vi "_RT Process Runtime Update.vi"(8 "Error In":errorcluster, 9 "Acquiring Data":bool, 10 "binary string":string, 11 "Command":T1) -> (0 "Error Out":errorcluster)   [LabVIEW 2015]
uses:
  Type/_RT Command.ctl
  Type/_RT Active Ch.ctl
  Type/_RT Parameter.ctl
  Type/_RT Expt.ctl
  Type/_Run Mode.ctl
  Type/_RT Mass Range.ctl
  Type/_RT Res Type.ctl
  _RT Global.vi
  <vilib>/Utility/error.llb/Error Cluster From Error Code.vi
  <vilib>/rvi/errors/niLvFpgaAdjustHostInterfaceError.vi
  <vilib>/rvi/interface/nirviReadWriteControl/nirviReadWriteControl.xnode
  Type/FPGA Typedef.ctl
  FPGA Bitfiles/FPGA9607.lvbitx
  NiFpgaLv.dll
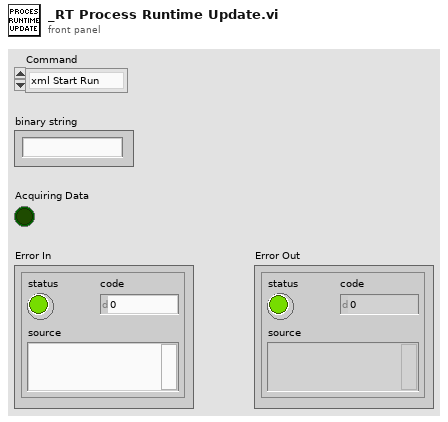
[diagram p1: front panel]
types:
  T1 = typedef "_RT Command.ctl" = enum16{"xml Start Run", "xml Start Actual Run", "xml Stop Run", "xml Runtime Update", "xml Get Status", "xml Get Table", "xml Set Table", "xml Get Configuration", "xml System Status", "xml Set LC Input Logic", "xml Get Data", "xml Get Info", "Start", "StartActualRun", "Stop", "Runtime Update", "Get Data", "Get Info", "Get Status", "Get Param", "Get Config", "Get Table", "Read ADC", "Set Oscillator", "Update Config", "Update Table", "Set All Pol", "Set Pol and DC", "Set Max Mass", "Toggle RP", "Toggle EL", "Set PIC", "Initialize Turbo", "Send Turbo Comm", "Close Turbo", "P1", "P2", "P3", "Send Serial", "Set LC Out", "Get LC In", "Read VAC", "Test Table", "Toggle Power", "Get Startup", "Set Startup", "Get ADC Table", "Set ADC Table", "Get Brief Status", "Get Detail Status", "Auxiliary Update", "Set CC Logics", "Set CC Input Logics", "Ignore Error", "invalid"}
  T2 = typedef "_RT Expt.ctl" = cluster{"StartT(mS)":i32, "#Cycles":i32, "Scan Type":T3, "PauseT(uS)":i32, "Polarity":u8, "DelayT(mS)":i32, "Active Ch":T4[], "Mass Range":T5[]}
  T3 = typedef "_Run Mode.ctl" = enum16{"MRM (Q1/Q2)", "Q1 Scan", "Q1 SRM", "Q2 Scan", "Q2 SRM", "Product Scan", "Precursor Scan", "Neutral Loss", "Neutral Gain"}
  T4 = typedef "_RT Active Ch.ctl" = cluster{"Start":i32, "Step":i32, "ChID":i32}
  T5 = typedef "_RT Mass Range.ctl" = cluster{"Steps":i32, "Dwell(uS)":i32, "Resolution Type":T6, "Ramping Ch":T4[]}
  T6 = typedef "_RT Res Type.ctl" = u16
  T7 = typedef "_RT Parameter.ctl" = cluster{"RunMode":i32, "Initial Ch":T4[], "Sync":u8, "Expt":T2[], "EqTime(mS)":i32}
  T8 = typedef "_RT Instrument State.ctl" = enum16{"Initializing", "Mass Spectrometer is Off", "Starting Up", "Turning Power Off", "Going to Standby", "Roughing Pump Ready", "Turning Turbo Off", "Turbo Startup", "Turbopump Ready", "Checking Vacuum", "Going to Ready", "Ready", "Running", "Source Standby", "Lost Communication", "Shutting Down", "Fault", "24V Standby", "Go to 24V Standby", "Turbopump Ready-Waiting"}
  T9 = typedef "Semaphore RefNum" = refnum<k1>
  T10 = typedef "_XML Lens.ctl" = cluster{"Value":dbl, "ChID":u8}
  T11 = typedef "FPGA Typedef.ctl" = refnum<k20>
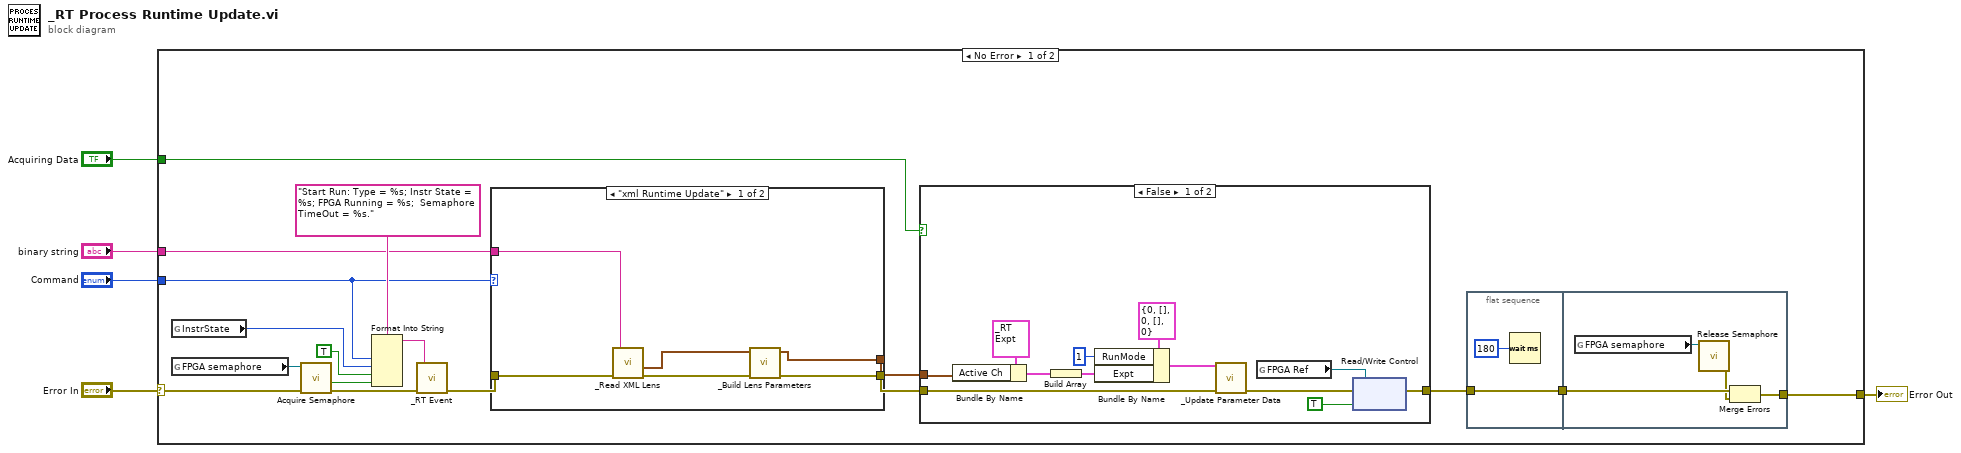
[diagram p0: block diagram]
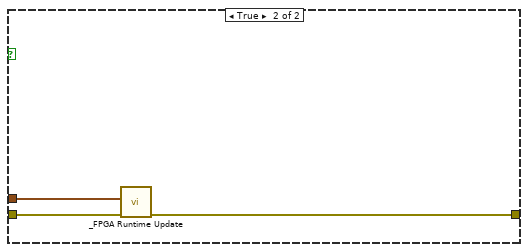
[diagram p2: hidden frame]
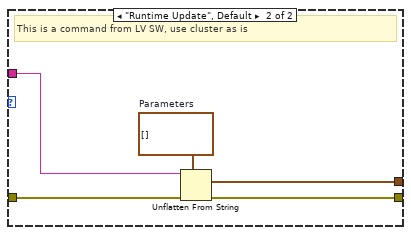
[diagram p3: hidden frame]
diagram:
  n1 = case shown="No Error" "Error In" {
    selector: "Error In" -> [w21 w55]
    tunnel: [w20 w55] -> w4
    tunnel: "Command" -> [w13 _]
    tunnel: "binary string" -> [w12 _]
    tunnel: "Acquiring Data" -> [w6 _]
    frame No Error {
      n2 = global read "_RT Global.vi" "InstrState"() -> (w8:T8)
      n3 = global read "_RT Global.vi" "FPGA semaphore"() -> (w16:T9)
      n4 = call <vilib>:"Acquire Semaphore.vi"("error in (no error)"=w21, "semaphore"=w16) -> ("error out"=w15:errorcluster, "timed out"=w17:bool)  [unwired: 1 in, 3 out]
      n5 = Format Into String(format string="Start Run: Type = %s; Instr State = %s; FPGA Running = %s;  Semaphore TimeOut = %s.", w13, w8, TRUE ("timed out"), w17) -> (resulting string=w18:string)  [unwired: 2 in, 1 out]
      n6 = call "_RT Event.vi"("error in (no error)"=w15, "Event"=w18) -> ("error out"=w14:errorcluster)  [unwired: 1 in, 4 out]
      n7 = case shown="\"xml Runtime Update\"" w13 {
        tunnel: [w46 w53] -> w11
        tunnel: w14 -> [w49 w54]
        tunnel: w12 -> [w48 w52]
        tunnel: [w44 w50] -> w10
        frame "xml Runtime Update" {
          n8 = call "_Read XML Lens.vi"("error in"=w49, "XML String"=w48) -> ("error out"=w47:errorcluster, "Lens"=w45:T10[])  [unwired: 4 out]
          n9 = call "_Build Lens Parameters.vi"("error in"=w47, "Lens"=w45) -> ("error out"=w46:errorcluster, "Array"=w44:T4[])  [unwired: 8 in]
        }
        frame "Runtime Update", Default {
          w51 = T4[] []  # Parameters
          # "This is a command from LV SW, use cluster as is"
          n10 = Unflatten From String(type=w51, binary string=w52, error in (no error)=w54) -> (value=w50:T4[], error out=w53:errorcluster)  [unwired: 3 out]
        }
      }
      n11 = case shown="False" w6 {
        tunnel: w11 -> [w27 w37]
        tunnel: w10 -> [w29 w36]
        tunnel: [w23 w35] -> w9
        frame False {
          n12 = Bundle By Name(cluster=T2 {"StartT(mS)"=0, "#Cycles"=0, "Scan Type"=enum."MRM (Q1/Q2)", "PauseT(uS)"=0, "Polarity"=0, "DelayT(mS)"=0, "Active Ch"=[], "Mass Range"=[]} ("Expt"), "Active Ch"=w29) -> (w32:T2)
          n13 = Build Array(w32) -> (w33:T2[])
          n14 = Bundle By Name(cluster=T7 {"RunMode"=0, "Initial Ch"=[], "Sync"=0, "Expt"=[], "EqTime(mS)"=0} ("Parameter"), "RunMode"=1, "Expt"=w33) -> (w28:T7)
          n15 = call "_Update Parameter Data.vi"("error in"=w27, "Parameter"=w28) -> ("error out"=w24:errorcluster)  [unwired: 1 in, 4 out]
          n16 = global read "_RT Global.vi" "FPGA Ref"() -> (w25:T11)
          n17 = xnode "Read/Write Control"("FPGA VI Reference In"=w25, "error in"=w24, "Start"=TRUE) -> ("error out"=w23:errorcluster)  [unwired: 1 out]
        }
        frame True {
          n18 = call "_FPGA Runtime Update.vi"("error in"=w37, "Parameters"=w36) -> ("error out"=w35:errorcluster)  [unwired: 1 in, 4 out]
        }
      }
      n19 = flat-sequence {
        tunnel: w9 -> [w39]
        tunnel: [w39] -> w22
        tunnel: [w42] -> w20
        tunnel: w22 -> [w43]
        frame #0 {
          n20 = Wait (ms)(milliseconds to wait=u32 180) -> ()  [unwired: 1 out]
        }
        frame #1 {
          n21 = global read "_RT Global.vi" "FPGA semaphore"() -> (w40:T9)
          n22 = call <vilib>:"Release Semaphore.vi"("semaphore"=w40) -> ("error out"=w41:errorcluster)  [unwired: 1 in, 5 out]
          n23 = Merge Errors(w43, w41) -> (w42:errorcluster)
        }
      }
    }
    frame Error {
    }
  }
  "Error Out" <- w4
